vi "LDT Ovservatory Status.vi"(11 "XML Locutus Obs Status String":string) -> (3 "keywords":T1[](array[typedef]))   [LabVIEW 2022 SP3, in "LDT Telescope.lvclass"]
uses:
  LDT Telescope.lvclass
  LDT FITS Keyword cluster.ctl
  <vilib>/regexp/Match Regular Expression.xnode
  LDT Telescope.lvclass/LDT Telescope.ctl
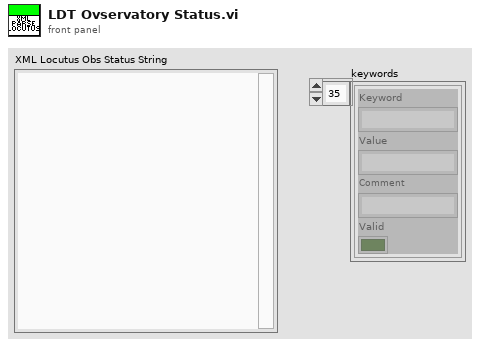
[diagram p1: front panel]
types:
  T1 = typedef "LDT Telescope.lvclass/LDT FITS Keyword cluster.ctl" = cluster{"Keyword":string, "Value":string, "Comment":string, "Valid":bool}
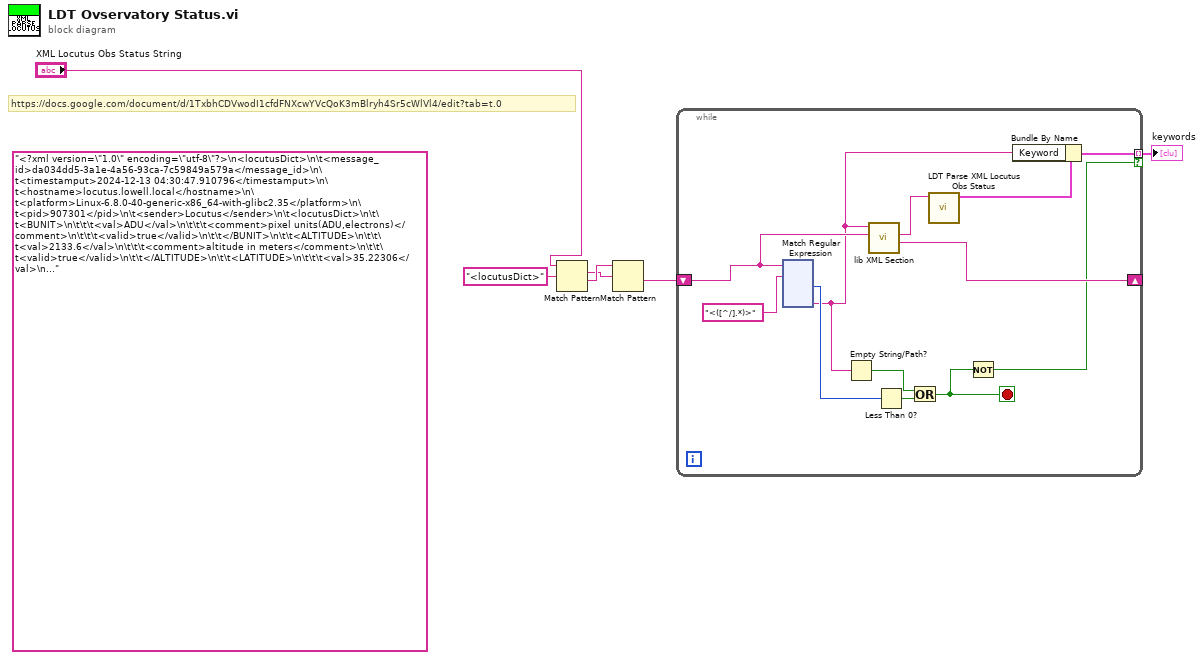
[diagram p0: block diagram]
diagram:
  (unwired) "<?xml version=\"1.0\" encoding=\"utf-8\"?>\n<locutusDict>\n\t<message_id>da034dd5-3a1e-4a56-93ca-7c59849a579a</message_id>\n\t<timestamput>2024-12-13 04:30:47.910796</timestamput>\n\t<hostname>locutus.lowell.local</hostname>\n\t<platform>Linux-6.8.0-40-generic-x86_64-with-glibc2.35</platform>\n\t<pid>907301</pid>\n\t<sender>Locutus</sender>\n\t<locutusDict>\n\t\t<BUNIT>\n\t\t\t<val>ADU</val>\n\t\t\t<comment>pixel units(ADU,electrons)</comment>\n\t\t\t<valid>true</valid>\n\t\t</BUNIT>\n\t\t<ALTITUDE>\n\t\t\t<val>2133.6</val>\n\t\t\t<comment>altitude in meters</comment>\n\t\t\t<valid>true</valid>\n\t\t</ALTITUDE>\n\t\t<LATITUDE>\n\t\t\t<val>35.22306</val>\n\t\t\t<comment>latitude, degrees</comment>\n\t\t\t<valid>true</valid>\n\t\t</LATITUDE>\n\t\t<LONGITUD>\n\t\t\t<val>-111.6025</val>\n\t\t\t<comment>east longitude, degrees</comment>\n\t\t\t<valid>true</valid>\n\t\t</LONGITUD>\n\t\t<DATUM>\n\t\t\t<val>WGS84</val>\n\t\t\t<comment>The coordinate system for longitude and latitude</comment>\n\t\t\t<valid>true</valid>\n\t\t</DATUM>\n\t\t<OBSREF>\n\t\t\t<val>WGS84</val>\n\t\t\t<comment>The coordinate system for longitude and latitude</comment>\n\t\t\t<valid>true</valid>\n\t\t</OBSREF>\n\t\t<FILENAME>\n\t\t\t<val>/data/testing/20241213/lbwr.20241213.00002.fits</val>\n\t\t\t<comment>Original Camera Disk Filename</comment>\n\t\t\t<valid>true</valid>\n\t\t</FILENAME>\n\t\t<OBSERNO>\n\t\t\t<val>2</val>\n\t\t\t<comment>Image Count for Observing Session</comment>\n\t\t\t<valid>true</valid>\n\t\t</OBSERNO>\n\t\t<OBJNAME>\n\t\t\t<val>Cube Frame Test</val>\n\t\t\t<comment>Target Object Name</comment>\n\t\t\t<valid>true</valid>\n\t\t</OBJNAME>\n\t\t<OBJECT>\n\t\t\t<val>Cube Frame Test</val>\n\t\t\t<comment>Object Name</comment>\n\t\t\t<valid>true</valid>\n\t\t</OBJECT>\n\t\t<OBSTYPE>\n\t\t\t<val>FOCUS</val>\n\t\t\t<comment>object, flat, bias, etc.</comment>\n\t\t\t<valid>true</valid>\n\t\t</OBSTYPE>\n\t\t<IMAGETYP>\n\t\t\t<val>FOCUS</val>\n\t\t\t<comment>object, flat, bias, etc.</comment>\n\t\t\t<valid>true</valid>\n\t\t</IMAGETYP>\n\t\t<CCDSUM>\n\t\t\t<val>1 1</val>\n\t\t\t<comment>On Chip binned summation</comment>\n\t\t\t<valid>true</valid>\n\t\t</CCDSUM>\n\t\t<DETTEMP>\n\t\t\t<val>14.7</val>\n\t\t\t<comment>CCD Temp in Deg C</comment>\n\t\t\t<valid>true</valid>\n\t\t</DETTEMP>\n\t\t<TEMPCCD>\n\t\t\t<val>14.7</val>\n\t\t\t<comment>CCD Temp in Deg C</comment>\n\t\t\t<valid>true</valid>\n\t\t</TEMPCCD>\n\t\t<SETTEMP>\n\t\t\t<val>15.0</val>\n\t\t\t<comment>CCD Temp Set Value in Deg C</comment>\n\t\t\t<valid>true</valid>\n\t\t</SETTEMP>\n\t\t<COOLPWR>\n\t\t\t<val>0.0</val>\n\t\t\t<comment>CCD Cooler power in %</comment>\n\t\t\t<valid>true</valid>\n\t\t</COOLPWR>\n\t\t<TEMPTOL>\n\t\t\t<val>15.0</val>\n\t\t\t<comment>CCD Temp diff from set value tolerance in Deg C</comment>\n\t\t\t<valid>true</valid>\n\t\t</TEMPTOL>\n\t\t<TELESCOP>\n\t\t\t<val>UNKNOWN</val>\n\t\t\t<comment>Telescope name</comment>\n\t\t\t<valid>true</valid>\n\t\t</TELESCOP>\n\t\t<LST-OBS>\n\t\t\t<val>02:33:48.290</val>\n\t\t\t<comment>Local Sidereal Time of exposure start</comment>\n\t\t\t<valid>true</valid>\n\t\t</LST-OBS>\n\t\t<TELRA>\n\t\t\t<val>02:32:16.110</val>\n\t\t\t<comment>TCS right ascension(hh:mm:ss)</comment>\n\t\t\t<valid>true</valid>\n\t\t</TELRA>\n\t\t<TELDEC>\n\t\t\t<val>+35:06:36.49</val>\n\t\t\t<comment>TCS declination (dd:mm:ss)</comment>\n\t\t\t<valid>true</valid>\n\t\t</TELDEC>\n\t\t<OBSRA>\n\t\t\t<val>02:32:16.110</val>\n\t\t\t<comment>requested right ascension(hh:mm:ss)</comment>\n\t\t\t<valid>true</valid>\n\t\t</OBSRA>\n\t\t<OBSDEC>\n\t\t\t<val>+35:06:36.49</val>\n\t\t\t<comment>requested declination (dd:mm:ss)</comment>\n\t\t\t<valid>true</valid>\n\t\t</OBSDEC>\n\t\t<AIRMASS>\n\t\t\t<val>1.0</val>\n\t\t\t<comment>airmass</comment>\n\t\t\t<valid>true</valid>\n\t\t</AIRMASS>\n\t\t<TELFOCUS>\n\t\t\t<val>UNKNOWN</val>\n\t\t\t<comment>telescope focus position</comment>\n\t\t\t<valid>true</valid>\n\t\t</TELFOCUS>\n\t\t<HA>\n\t\t\t<val>00:01:32.179</val>\n\t\t\t<comment>hour angle</comment>\n\t\t\t<valid>true</valid>\n\t\t</HA>\n\t\t<ZA>\n\t\t\t<val>0.0</val>\n\t\t\t<comment>zenith angle</comment>\n\t\t\t<valid>true</valid>\n\t\t</ZA>\n\t\t<ZD>\n\t\t\t<val>0.0</val>\n\t\t\t<comment>zenith angle</comment>\n\t\t\t<valid>true</valid>\n\t\t</ZD>\n\t\t<PARANGLE>\n\t\t\t<val>70.1081</val>\n\t\t\t<comment>Parallactic Angle at start of exposure</comment>\n\t\t\t<valid>true</valid>\n\t\t</PARANGLE>\n\t\t<RA>\n\t\t\t<val>02:32:16.110</val>\n\t\t\t<comment>Right Ascension</comment>\n\t\t\t<valid>true</valid>\n\t\t</RA>\n\t\t<DEC>\n\t\t\t<val>+35:06:36.49</val>\n\t\t\t<comment>Declination</comment>\n\t\t\t<valid>true</valid>\n\t\t</DEC>\n\t\t<ST>\n\t\t\t<val>02:33:48.290</val>\n\t\t\t<comment>Local Sidereal Time</comment>\n\t\t\t<valid>true</valid>\n\t\t</ST>\n\t\t<TELALT>\n\t\t\t<val>0.0</val>\n\t\t\t<comment>Telescope Altitude at start of exposure</comment>\n\t\t\t<valid>true</valid>\n\t\t</TELALT>\n\t\t<TELAZ>\n\t\t\t<val>0.0</val>\n\t\t\t<comment>Telescope Azimuth at start of exposure</comment>\n\t\t\t<valid>true</valid>\n\t\t</TELAZ>\n\t\t<KWDICT>\n\t\t\t<val>ldtboresight_wr v0.1</val>\n\t\t\t<comment>FITS keyword dictionary - 2024 Feb 14</comment>\n\t\t\t<valid>true</valid>\n\t\t</KWDICT>\n\t\t<OBSLAT>\n\t\t\t<val>35.22306</val>\n\t\t\t<comment>Observatory Latitude (degrees)</comment>\n\t\t\t<valid>true</valid>\n\t\t</OBSLAT>\n\t\t<OBSLONG>\n\t\t\t<val>-111.6025</val>\n\t\t\t<comment>Observatory Longitude (degrees)</comment>\n\t\t\t<valid>true</valid>\n\t\t</OBSLONG>\n\t\t<OBSALT>\n\t\t\t<val>2133.6</val>\n\t\t\t<comment>Observatory Altitude (meters)</comment>\n\t\t\t<valid>true</valid>\n\t\t</OBSALT>\n\t\t<INSTRUME>\n\t\t\t<val>ZWO CCD ASI6200MM Pro</val>\n\t\t\t<comment>Instrument</comment>\n\t\t\t<valid>true</valid>\n\t\t</INSTRUME>\n\t\t<FILTERS>\n\t\t\t<val>SDSS-R</val>\n\t\t\t<comment>Filter Name</comment>\n\t\t\t<valid>true</valid>\n\t\t</FILTERS>\n\t</locutusDict>\n</locutusDict>\n\n"
  # "https://docs.google.com/document/d/1TxbhCDVwodI1cfdFNXcwYVcQoK3mBlryh4Sr5cWlVl4/edit?tab=t.0"
  n1 = Match Pattern(string="XML Locutus Obs Status String", regular expression="<locutusDict>") -> (match substring=w4:string, after substring=w5:string)  [unwired: 1 in, 2 out]
  n2 = Match Pattern(string=w5, regular expression=w4) -> (after substring=w3:string)  [unwired: 1 in, 3 out]
  n3 = while {
    shift-right: [w13] -> _
    shift-left: w3 -> [w14]
    tunnel: [w9] -> w2 mode=indexing if=w7
    stop <- w8 stop-if-true
    n4 = xnode "Match Regular Expression"("input string"=w14, "regular expression"="<([^/].*)>") -> ("offset past match"=w17:i32, "submatch 1"=w10:string)  [unwired: 4 in, 4 out]
    n5 = Empty String/Path?(string/path=w10) -> (empty?=w15:bool)
    n6 = call "lib XML Section.vi"("XML String"=w14, "XML Topic"=w10) -> ("after substring"=w13:string, "XML Topic Body"=w12:string)  [unwired: 6 in, 2 out]
    n7 = Less Than 0?(x=w17) -> (x < 0?=w16:bool)
    n8 = Or(x=w15, y=w16) -> (x .or. y?=w8:bool)
    n9 = call "LDT Parse XML Locutus Obs Status.vi"("XML String"=w12) -> ("FITS Keyword"=w11:T1)  [unwired: 10 in]
    n10 = Not(x=w8) -> (.not. x?=w7:bool)
    n11 = Bundle By Name(cluster=w11, "Keyword"=w10) -> (w9:T1)
  }
  "keywords" <- w2
